vi "test_IncrementalBuild_SplitProjectTargetsSolution.vi"() -> (3 "Pass?":bool)   [LabVIEW 2019, in "Tests.SolutionBuilder.lvlib"]
uses:
  Tests.SolutionBuilder.lvlib
  SolutionBuilder/SolutionBuilder.lvclass
panel:
  out "Second build":cluster{"Build spec name":string, "size":i32}[](array[cluster])
  out "First build":cluster{"Build spec name":string, "size":i32}[](array[cluster])
  out "error out":errorcluster
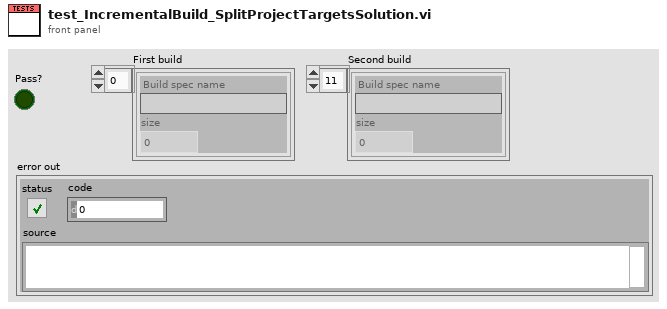
[diagram p1: front panel]
types:
  T1 = typedef "SolutionBuilder.lvlib/BuildManager.lvclass/GeneratedFile.ctl" = map{cluster{"Project path":string, "Build spec name":string}, set{string}}
  T2 = cluster{"Project path":string, "Build spec name":string}
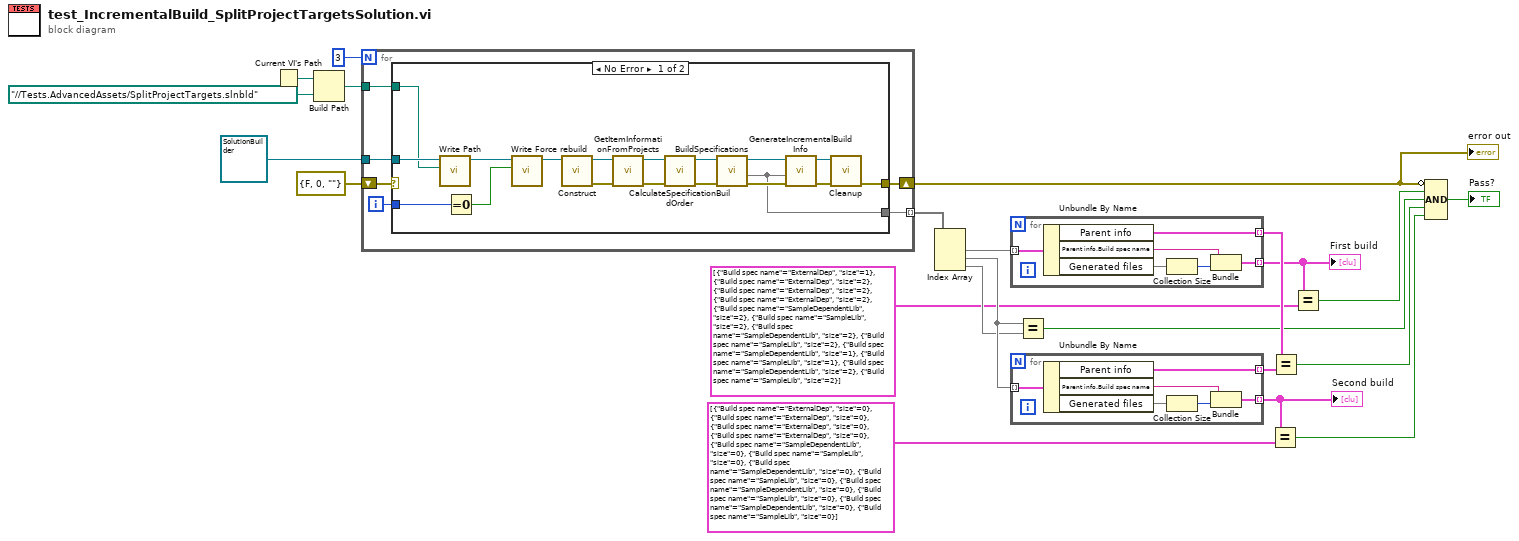
[diagram p0: block diagram]
diagram:
  n1 = Current VI's Path() -> (path=w20:path)
  n2 = Build Path(base path=w20, name or relative path=path "../../Tests.AdvancedAssets/SplitProjectTargets.slnbld" ("Path")) -> (appended path=w18:path)
  n3 = for {
    N: 3 -> [_]
    tunnel: refnum<class "SolutionBuilder.lvclass"> refnum ("SolutionBuilder in") -> [w27]
    tunnel: w18 -> [w25]
    shift-right: [w28] -> w22
    shift-left: errorcluster {"status"=FALSE, "code"=0, "source"=""} ("error IO") -> [w26]
    tunnel: [w24] -> w17 mode=indexing
    i -> [w23]
    n4 = case shown="No Error" w26 {
      selector: w26 -> [_ w47]
      tunnel: w27 -> [w40 _]
      tunnel: [w39 w47] -> w28
      tunnel: w25 -> [w38 _]
      tunnel: [w31 _] -> w24
      tunnel: w23 -> [w35 _]
      frame No Error {
        n5 = call "Write Path.vi"("Path"=w38, "SolutionBuilder in"=w40) -> ("SolutionBuilder out"=w37:refnum<class "SolutionBuilder.lvclass">)  [unwired: 9 in]
        n6 = Equal To 0?(x=w35) -> (x = 0?=w34:bool)
        n7 = call "Write Force rebuild.vi"("Force rebuild"=w34, "SolutionBuilder in"=w37) -> ("SolutionBuilder out"=w36:refnum<class "SolutionBuilder.lvclass">)  [unwired: 9 in]
        n8 = call "Construct.vi"("SolutionBuilder in"=w36) -> ("error out"=w44:errorcluster, "SolutionBuilder out"=w41:refnum<class "SolutionBuilder.lvclass">)  [unwired: 9 in]
        n9 = call "GetItemInformationFromProjects.vi"("error in (no error)"=w44, "SolutionBuilder in"=w41) -> ("error out"=w45:errorcluster, "SolutionBuilder out"=w42:refnum<class "SolutionBuilder.lvclass">)  [unwired: 8 in]
        n10 = call "CalculateSpecificationBuildOrder.vi"("error in (no error)"=w45, "SolutionBuilder in"=w42) -> ("error out"=w46:errorcluster, "SolutionBuilder out"=w43:refnum<class "SolutionBuilder.lvclass">)  [unwired: 8 in]
        n11 = call "BuildSpecifications.vi"("error in (no error)"=w46, "SolutionBuilder in"=w43) -> ("error out"=w32:errorcluster, "Generated file"=w31:T1, "SolutionBuilder out"=w33:refnum<class "SolutionBuilder.lvclass">)  [unwired: 7 in]
        n12 = call "GenerateIncrementalBuildInfo.vi"("error in (no error)"=w32, "Generated file"=w31, "SolutionBuilder in"=w33) -> ("error out"=w29:errorcluster, "SolutionBuilder out"=w30:refnum<class "SolutionBuilder.lvclass">)  [unwired: 7 in]
        n13 = call "Cleanup.vi"("error in (no error)"=w29, "SolutionBuilder in"=w30) -> ("error out"=w39:errorcluster)  [unwired: 8 in, 1 out]
      }
      frame Error {
      }
    }
  }
  "error out" <- w22
  n14 = Index Array(array=w17) -> (element #1=w16:T1, element #2=w5:T1, element #3=w4:T1)  [unwired: 3 in]
  n15 = for {
    tunnel: w16 -> [w53] mode=indexing
    tunnel: [w52] -> w15 mode=indexing
    tunnel: [w48] -> w12 mode=indexing
    n16 = Unbundle By Name(w53) -> ("Parent info"=w52:T2, "Parent info.Build spec name"=w50:string, "Generated files"=w51:set{string})
    n17 = Collection Size(1:w51) -> (0:w49:i32)
    n18 = Bundle("Build spec name"=w50, "size"=w49) -> (w48:cluster{"Build spec name":string, "size":i32})  [unwired: 1 in]
  }
  "First build" <- w12
  n19 = for {
    tunnel: w5 -> [w59] mode=indexing
    tunnel: [w58] -> w13 mode=indexing
    tunnel: [w54] -> w9 mode=indexing
    n20 = Unbundle By Name(w59) -> ("Parent info"=w58:T2, "Parent info.Build spec name"=w56:string, "Generated files"=w57:set{string})
    n21 = Collection Size(1:w57) -> (0:w55:i32)
    n22 = Bundle("Build spec name"=w56, "size"=w55) -> (w54:cluster{"Build spec name":string, "size":i32})  [unwired: 1 in]
  }
  "Second build" <- w9
  n23 = Equal?(x=w5, y=w4) -> (x = y?=w3:bool)
  n24 = Equal?(x=w9, y=cluster{"Build spec name":string, "size":i32}[] [{"Build spec name"="ExternalDep", "size"=0}, {"Build spec name"="ExternalDep", "size"=0}, {"Build spec name"="ExternalDep", "size"=0}, {"Build spec name"="ExternalDep", "size"=0}, {"Build spec name"="SampleDependentLib", "size"=0}, {"Build spec name"="SampleLib", "size"=0}, {"Build spec name"="SampleDependentLib", "size"=0}, {"Build spec name"="SampleLib", "size"=0}, {"Build spec name"="SampleDependentLib", "size"=0}, {"Build spec name"="SampleLib", "size"=0}, {"Build spec name"="SampleDependentLib", "size"=0}, {"Build spec name"="SampleLib", "size"=0}] ("Second build")) -> (x = y?=w8:bool)
  n25 = Equal?(x=w15, y=w13) -> (x = y?=w11:bool)
  n26 = Equal?(x=w12, y=cluster{"Build spec name":string, "size":i32}[] [{"Build spec name"="ExternalDep", "size"=1}, {"Build spec name"="ExternalDep", "size"=2}, {"Build spec name"="ExternalDep", "size"=2}, {"Build spec name"="ExternalDep", "size"=2}, {"Build spec name"="SampleDependentLib", "size"=2}, {"Build spec name"="SampleLib", "size"=2}, {"Build spec name"="SampleDependentLib", "size"=2}, {"Build spec name"="SampleLib", "size"=2}, {"Build spec name"="SampleDependentLib", "size"=1}, {"Build spec name"="SampleLib", "size"=1}, {"Build spec name"="SampleDependentLib", "size"=2}, {"Build spec name"="SampleLib", "size"=2}] ("First build")) -> (x = y?=w10:bool)
  n27 = Compound Arithmetic op=AND(invert w22, w10, w3, w11, w8) -> (→"Pass?":bool)
